vi "Display and Log Process.vi"(10 "Parameters":variant, 11 "Process":refnum<class "Process.lvclass">) -> ()   [LabVIEW 2015, in "VS Inline Async API.lvlib"]
uses:
  VS Inline Async API.lvlib
  Process/Process.lvclass
  Process/Process.lvclass/Process.ctl
  Process/Data Member Access/Read Name.vi
  Process/Data Member Access/Read Process.Trigger.vi
  Process/Data Member Access/Read Process.Stop.vi
  SubVIs/Error.Message.Format.vi
  SubVIs/Error.Tags.Check.vi
  <vilib>/Utility/error.llb/Find Tag.vi
  <vilib>/Utility/error.llb/Trim Whitespace.vi
  <vilib>/Utility/error.llb/Error Code Database.vi
  <vilib>/NI Veristand/Custom Device Tools/Custom Device Utility Library/Custom Device Utility Library.lvlib
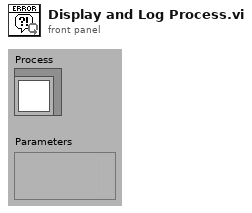
[diagram p1: front panel]
types:
  T1 = cluster{"read mode":enum16{"polling", "blocking"}, "write mode":enum16{"polling", "blocking"}}
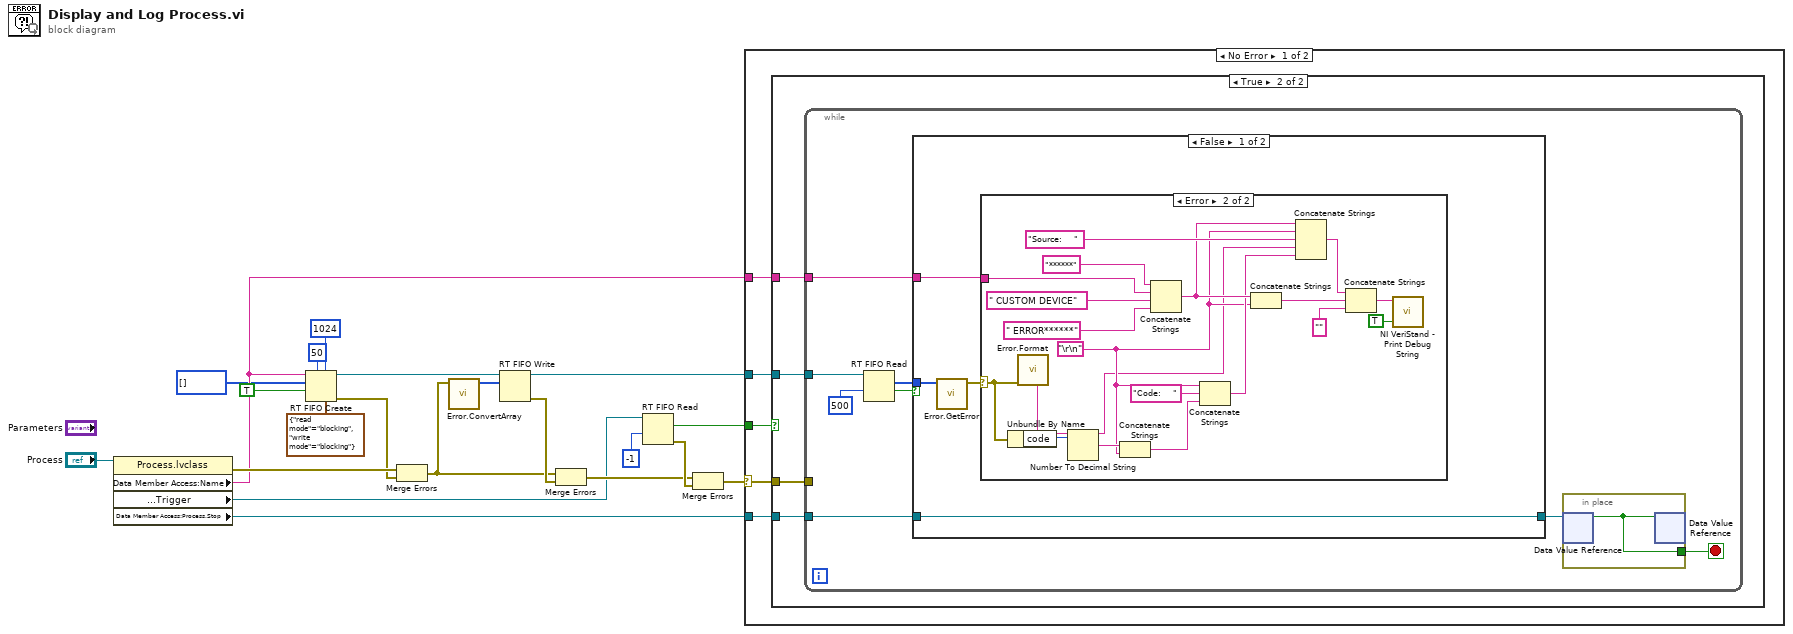
[diagram p0: block diagram]
diagram:
  n1 = property class="Process.lvclass"(reference="Process") -> (error out=w18:errorcluster, "Data Member Access:Name"=w16:string, "Data Member Access:Process.Trigger"=w3:refnum<k33>, "Data Member Access:Process.Stop"=w19:refnum<data-value>)  [unwired: 1 in, 1 out]
  n2 = RT FIFO Create(0:w16, 1:u8[] [], 2:TRUE ("create if not found? (T)"), 4:u32 50 ("size (10)"), 6:u32 1024 ("elements in array (1)"), 7:T1 {"read mode"=enum."blocking", "write mode"=enum."blocking"} ("r/w modes (polling,polling)")) -> (8:w21:refnum<k33>, 11:w15:errorcluster)  [unwired: 2 in, 1 out]
  n3 = Merge Errors(w18, w15) -> (w14:errorcluster)
  n4 = call "Error.ConvertArray.vi"("error in"=w14) -> ("Msg"=w11:u8[])  [unwired: 10 in]
  n5 = RT FIFO Write(0:w21, 1:w11) -> (8:w1:refnum<k33>, 11:w17:errorcluster)  [unwired: 3 in, 2 out]
  n6 = Merge Errors(w14, w17) -> (w5:errorcluster)
  n7 = RT FIFO Read(0:w3, 2:-1 ("timeout in ms (-1)")) -> (9:w2:bool, 11:w6:errorcluster)  [unwired: 2 in, 3 out]
  n8 = Merge Errors(w5, w6) -> (w4:errorcluster)
  n9 = case shown="No Error" w4 {
    selector: w4 -> [w22 _]
    tunnel: w2 -> [w26 _]
    tunnel: w16 -> [w25 _]
    tunnel: w1 -> [w24 _]
    tunnel: w19 -> [w23 _]
    frame No Error {
      n10 = case shown="True" w26 {
        tunnel: w24 -> [_ w30]
        tunnel: w25 -> [_ w29]
        tunnel: w22 -> [_ w28]
        tunnel: w23 -> [_ w27]
        frame False {
        }
        frame True {
          n11 = while {
            tunnel: w30 -> [w38]
            tunnel: w29 -> [w37]
            tunnel: w28 -> [_]
            tunnel: w27 -> [w31]
            stop <- w33 stop-if-true
            n12 = RT FIFO Read(0:w38, 2:500 ("timeout in ms (-1)")) -> (9:w36:u8[], 10:w34:bool)  [unwired: 2 in, 3 out]
            n13 = case shown="False" w34 {
              tunnel: w36 -> [w42 _]
              tunnel: w37 -> [w41 _]
              tunnel: [w43 w63] -> w32
              tunnel: w31 -> [w43 w63]
              frame False {
                n14 = call "Error.GetError.vi"("Msg"=w42) -> ("error out"=w40:errorcluster)  [unwired: 10 in]
                n15 = case shown="Error" w40 {
                  selector: w40 -> [_ w45]
                  tunnel: w41 -> [_ w50]
                  frame No Error {
                  }
                  frame Error {
                    w49 = "\r\n"
                    n16 = Unbundle By Name(w45) -> ("code"=w52:i32)
                    n17 = call "Error.Format.vi"("error in (no error)"=w45) -> ("message"=w44:string)  [unwired: 6 in, 4 out]
                    n18 = Number To Decimal String(number=w52) -> (decimal integer string=w60:string)  [unwired: 1 in]
                    n19 = Concatenate Strings(w60, w49) -> (w51:string)
                    n20 = Concatenate Strings("******" ("String"), w50, " CUSTOM DEVICE" ("String"), " ERROR******" ("String")) -> (w57:string)
                    n21 = Concatenate Strings(w49, "Code:    " ("String"), w51) -> (w56:string)
                    n22 = Concatenate Strings(w57, w49) -> (w54:string)
                    n23 = Concatenate Strings(w57, w49, "Source:    " ("String"), w44, w56) -> (w55:string)
                    n24 = Concatenate Strings(w55, w54, "" ("Message")) -> (w48:string)
                    n25 = call <vilib>:"NI VeriStand - Print Debug String.vi"("Add to log file? (T)"=TRUE, "Message"=w48) -> ()  [unwired: 9 in, 1 out]
                  }
                }
              }
              frame True {
              }
            }
            n26 = in-place {
              in-place-border: [w39] -> w33
              n27 = in-place-dvr #1(w32) -> (w39:bool)  [unwired: 1 out]
              n28 = in-place-dvr #1(w39) -> ()  [unwired: 2 out]
            }
          }
        }
      }
    }
    frame Error {
    }
  }
